vi "get channel names from typedef.vi"(8 "error in":errorcluster, 11 "channel classification":T1) -> (0 "error out":errorcluster, 3 "Channel Names":string[](array[string]))   [LabVIEW 2013, in "fixed channel tag bus module configuration.lvclass"]
uses:
  fixed channel tag bus module configuration.lvclass
  <vilib>/NI/Tag Bus Module Framework/channel/channel classification.ctl
  execution/Runtime data typedefs/inputs.ctl
  execution/Runtime data typedefs/outputs.ctl
  execution/Runtime data typedefs/parameters.ctl
  execution/Runtime data typedefs/results.ctl
  execution/fixed channel tag bus module.lvclass
  <vilib>/Utility/VariantDataType/VariantType.lvlib
  <vilib>/NI/Tag Bus Module Framework/channel/TBM channel.lvclass
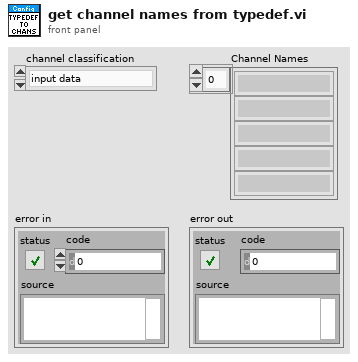
[diagram p1: front panel]
types:
  T1 = typedef "TBM channel.lvclass/channel classification.ctl" = enum16{"input data", "output data", "processing parameter", "processing result"}
  T2 = typedef "fixed channel tag bus module.lvclass/inputs.ctl" = cluster{"placeholder":i32}
  T3 = typedef "fixed channel tag bus module.lvclass/outputs.ctl" = cluster{"placeholder":i32}
  T4 = typedef "fixed channel tag bus module.lvclass/parameters.ctl" = cluster{"placeholder":i32}
  T5 = typedef "fixed channel tag bus module.lvclass/results.ctl" = cluster{"placeholder":i32}
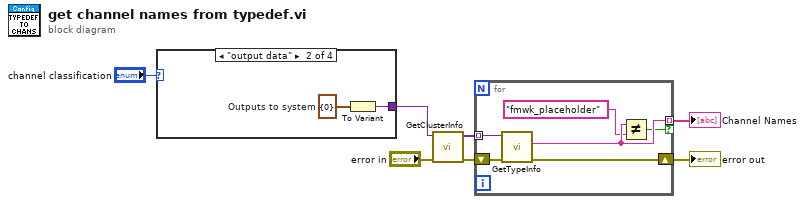
[diagram p0: block diagram]
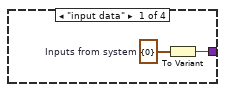
[diagram p2: hidden frame]
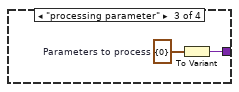
[diagram p3: hidden frame]
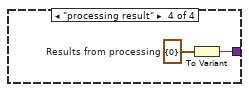
[diagram p4: hidden frame]
diagram:
  n1 = case shown="\"output data\"" "channel classification" {
    tunnel: [w8 w10 w13 w14] -> w3
    frame "input data" {
      w9 = T2 {"placeholder"=0}  # Inputs from system
      n2 = To Variant(anything=w9) -> (Variant=w8:variant)
    }
    frame "output data" {
      w11 = T3 {"placeholder"=0}  # Outputs to system
      n3 = To Variant(anything=w11) -> (Variant=w10:variant)
    }
    frame "processing parameter" {
      w12 = T4 {"placeholder"=0}  # Parameters to process
      n4 = To Variant(anything=w12) -> (Variant=w13:variant)
    }
    frame "processing result" {
      w15 = T5 {"placeholder"=0}  # Results from processing
      n5 = To Variant(anything=w15) -> (Variant=w14:variant)
    }
  }
  n6 = call <vilib>:"GetClusterInfo.vi"("error in (no error)"="error in", "Variant"=w3) -> ("error out"=w5:errorcluster, "Cluster Elements"=w6:variant[])  [unwired: 8 in]
  n7 = for {
    tunnel: w6 -> [w21] mode=indexing
    tunnel: [w18] -> w1 mode=indexing if=w17
    shift-right: [w20] -> w2
    shift-left: w5 -> [w19]
    n8 = call <vilib>:"GetTypeInfo.vi"("error in (no error)"=w19, "Variant"=w21) -> ("error out"=w20:errorcluster, "Name"=w18:string)  [unwired: 5 in, 3 out]
    n9 = Not Equal?(x=w18, y="fmwk_placeholder") -> (x != y?=w17:bool)
  }
  "Channel Names" <- w1
  "error out" <- w2
